vi "TestMode_RangeValidation.vi"(4 "TestAmplitudeLoopC1":i32, 5 "TestAmplitude":i32, 6 "TestAmplitudeLoopC2":i32, 7 "TestFrequencyLow":i32, 9 "TestPhaseLoopI":i32, 10 "TestPhaseLoopCF":i32, 11 "TestFrequencyHigh":i32) -> (3 "String":string)   [LabVIEW 2017]
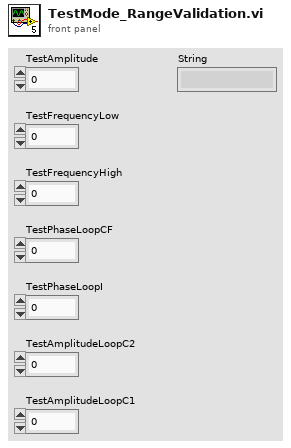
[diagram p1: front panel]
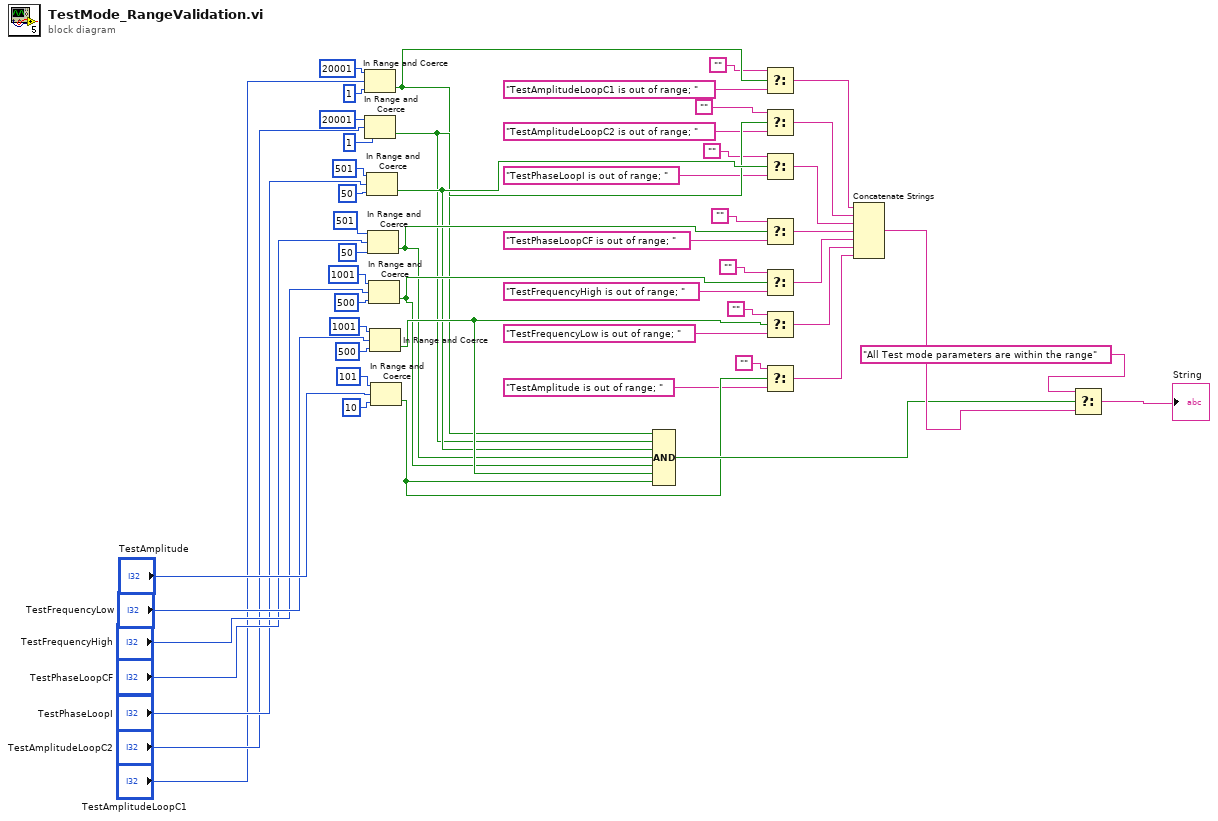
[diagram p0: block diagram]
diagram:
  n1 = In Range and Coerce(upper limit=20001, x="TestAmplitudeLoopC1", lower limit=1) -> (In Range?=w43:bool)  [unwired: 1 out]
  n2 = In Range and Coerce(upper limit=20001, x="TestAmplitudeLoopC2", lower limit=1) -> (In Range?=w44:bool)  [unwired: 1 out]
  n3 = In Range and Coerce(upper limit=501, x="TestPhaseLoopI", lower limit=50) -> (In Range?=w45:bool)  [unwired: 1 out]
  n4 = In Range and Coerce(upper limit=501, x="TestPhaseLoopCF", lower limit=50 ("x")) -> (In Range?=w46:bool)  [unwired: 1 out]
  n5 = In Range and Coerce(upper limit=1001, x="TestFrequencyHigh", lower limit=500) -> (In Range?=w47:bool)  [unwired: 1 out]
  n6 = In Range and Coerce(upper limit=1001, x="TestFrequencyLow", lower limit=500) -> (In Range?=w48:bool)  [unwired: 1 out]
  n7 = In Range and Coerce(upper limit=101, x="TestAmplitude", lower limit=10) -> (In Range?=w49:bool)  [unwired: 1 out]
  n8 = Compound Arithmetic op=AND(w43, w44, w45, w46, w47, w48, w49) -> (w50:bool)
  n9 = Select(t="", s=w43, f="TestAmplitudeLoopC1 is out of range; ") -> (s? t:f=w36:string)
  n10 = Select(t="", s=w44, f="TestAmplitudeLoopC2 is out of range; ") -> (s? t:f=w37:string)
  n11 = Select(t="", s=w45, f="TestPhaseLoopI is out of range; ") -> (s? t:f=w38:string)
  n12 = Select(t="", s=w46, f="TestPhaseLoopCF is out of range; ") -> (s? t:f=w39:string)
  n13 = Select(t="", s=w47, f="TestFrequencyHigh is out of range; ") -> (s? t:f=w40:string)
  n14 = Select(t="", s=w48, f="TestFrequencyLow is out of range; ") -> (s? t:f=w41:string)
  n15 = Select(t="", s=w49, f="TestAmplitude is out of range; ") -> (s? t:f=w42:string)
  n16 = Concatenate Strings(w36, w37, w38, w39, w40, w41, w42) -> (w51:string)
  n17 = Select(t="All Test mode parameters are within the range", s=w50, f=w51) -> (s? t:f=→"String":string)
